vi "setCrosstalkThreshold.vi"(0 "connection ID":refnum<k5>, 1 "axis":i32, 2 "threshold":i32, 3 "slipphasetime":i32, 5 "error":errorcluster) -> (14 "connection ID out":refnum<k5>, 15 "axis_out":i32, 19 "error out":errorcluster)   [LabVIEW 2016, in "amc_api.lvlib"]
doc: "This function sets the threshold range to avoid axis-crosstalk and slip phase time which is used while moving another axis"
uses:
  amc_api.lvlib
panel:
  out "jsonRespIn":string
  out "JSON-response":string="{\"jsonrpc\":\"2.0\",\"method\":\"\",\"params\":[5,1.245,true,\"name\"],\"id\":\"1\"}"
  out "JSON request":string
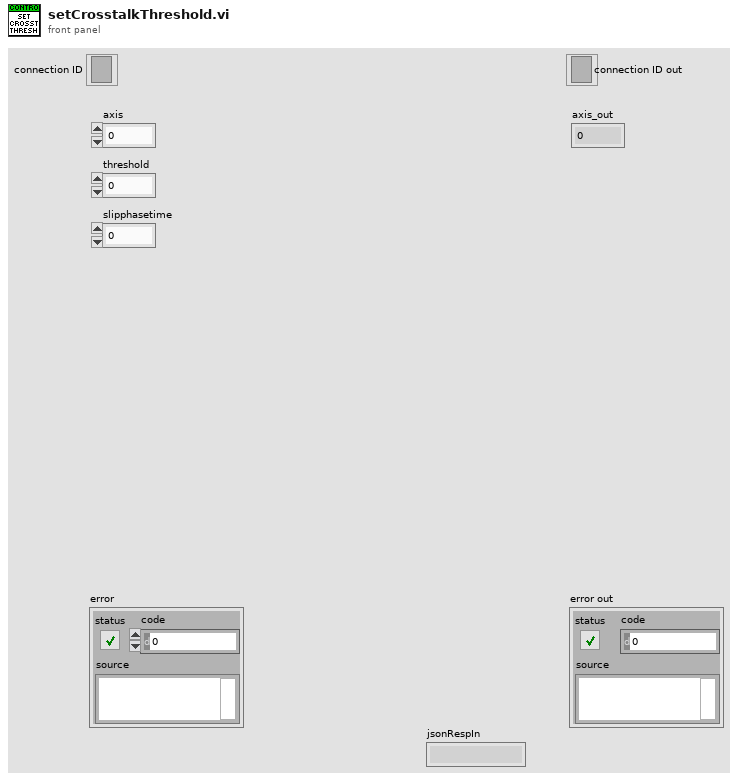
[diagram p1: front panel]
types:
  T1 = cluster{"jsonrpc":string, "method":string, "params":string[], "id":string, "api":i32, "pid":string}
  T2 = enum16{"Standard", "Buffered", "CRLF", "Immediate"}
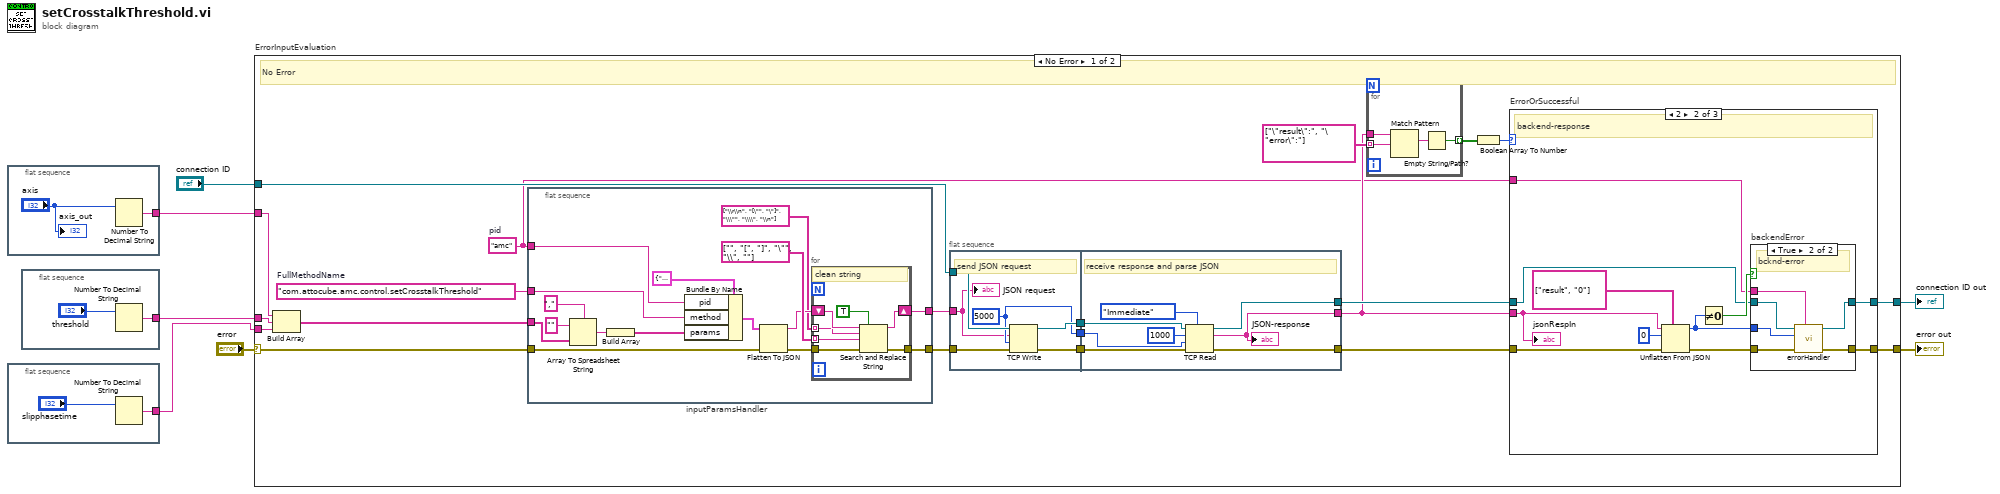
[diagram p0: block diagram]
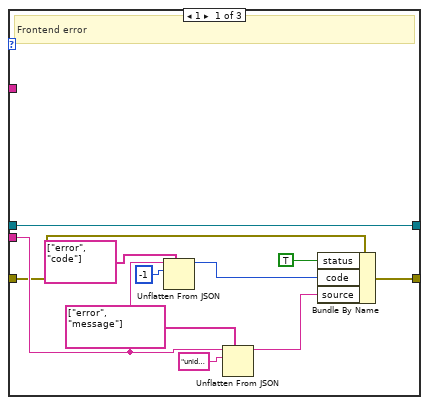
[diagram p2: hidden frame]
diagram:
  n1 = flat-sequence "in_axis" {
    tunnel: [w9] -> w3
    frame #0 {
      n2 = Number To Decimal String(number="axis") -> (decimal integer string=w9:string)  [unwired: 1 in]
      "axis_out" <- "axis"
    }
  }
  n3 = flat-sequence "in_integer" {
    tunnel: [w10] -> w1
    frame #0 {
      n4 = Number To Decimal String(number="slipphasetime") -> (decimal integer string=w10:string)  [unwired: 1 in]
    }
  }
  n5 = flat-sequence "in_integer" {
    tunnel: [w12] -> w2
    frame #0 {
      n6 = Number To Decimal String(number="threshold") -> (decimal integer string=w12:string)  [unwired: 1 in]
    }
  }
  n7 = case "ErrorInputEvaluation" shown="No Error" "error" {
    selector: "error" -> [w27 w108]
    tunnel: "connection ID" -> [w31 w109]
    tunnel: [w18 w108] -> w6
    tunnel: [w19 w109] -> w5
    tunnel: w3 -> [w16 _]
    tunnel: w2 -> [w15 _]
    tunnel: w1 -> [w14 _]
    frame No Error {
      w17 = "amc"  # pid
      w28 = "com.attocube.amc.control.setCrosstalkThreshold"  # FullMethodName
      # "No Error"
      n8 = Build Array ("ParametersArrayString")(w16, w15, w14) -> (w26:string[])
      n9 = flat-sequence "inputParamsHandler" {
        tunnel: [w72] -> w25
        tunnel: w26 -> [w78]
        tunnel: w27 -> [w77]
        tunnel: [w74] -> w24
        tunnel: w28 -> [w68]
        tunnel: w17 -> [w67]
        frame #0 {
          n10 = Array To Spreadsheet String(delimiter (Tab)=",", array=w78, 3:"" ("format string")) -> (spreadsheet string=w80:string)
          n11 = Build Array "Build Array"(w80) -> (w69:string[])
          n12 = Bundle By Name(cluster=T1 {"jsonrpc"="2.0", "method"="com.attocube.amc.res.setRESReadOutFreq", "params"=[], "id"="1", "api"=2, "pid"=""} ("Cluster"), "pid"=w67, "method"=w68, "params"=w69) -> (w79:T1)
          n13 = Flatten To JSON(anything=w79, error in (no error)=w77) -> (JSON string=w73:string, 11:w75:errorcluster)  [unwired: 1 in]
          n14 = for {
            tunnel: string[] ["\\r\\n", "[\"", "\"]", "\\\"", "\\\\", "\\n"] ("search string") -> [w86] mode=indexing
            tunnel: string[] ["", "[", "]", "\"", "\\", ""] ("replace string (\"\")") -> [w85] mode=indexing
            shift-right: [w88] -> w72
            shift-left: w73 -> [w87]
            tunnel: w75 -> [w84]
            tunnel: [w83] -> w74
            # "clean string"
            n15 = Search and Replace String(replace all?=TRUE ("replace all? (F)"), input string=w87, search string=w86, replace string=w85, error in=w84) -> (result string=w88:string, error out=w83:errorcluster)  [unwired: 3 in, 2 out]
          }
        }
      }
      n16 = flat-sequence {
        tunnel: w31 -> [w99]
        tunnel: [w97] -> w34
        tunnel: [w98] -> w33
        tunnel: w24 -> [w94]
        tunnel: [w96] -> w32
        tunnel: w25 -> [w95]
        tunnel: [w103] -> w23
        tunnel: w34 -> [w105]
        tunnel: w33 -> [w104]
        tunnel: [w101] -> w22
        tunnel: w32 -> [w102]
        tunnel: [w100] -> w21
        frame #0 {
          w96 = 5000 ("timeout ms (25000)")
          # "send JSON request"
          n17 = TCP Write(connection ID=w99, data in=w95, error in (no error)=w94, 9:w96) -> (connection ID out=w97:refnum<k5>, error out=w98:errorcluster)  [unwired: 1 out]
          "JSON request" <- w95
        }
        frame #1 {
          # "receive response and parse JSON"
          n18 = TCP Read(connection ID=w105, bytes to read=1000, error in (no error)=w104, 7:T2."Immediate" ("mode (standard)"), 9:w102) -> (connection ID out=w103:refnum<k5>, data out=w100:string, error out=w101:errorcluster)
          "JSON-response" <- w100
        }
      }
      n19 = for {
        tunnel: string[] ["\"result\":", "\"error\":"] ("path") -> [w92] mode=indexing
        tunnel: [w90] -> w29 mode=indexing
        tunnel: w21 -> [w93]
        n20 = Match Pattern(string=w93, regular expression=w92) -> (match substring=w91:string)  [unwired: 1 in, 3 out]
        n21 = Empty String/Path?(string/path=w91) -> (empty?=w90:bool)
      }
      n22 = Boolean Array To Number(Boolean array=w29) -> (number=w20:u32)
      n23 = case "ErrorOrSuccessful" shown="2" w20 {
        tunnel: w21 -> [w37 w48 _]
        tunnel: w23 -> [w35 w50 w66]
        tunnel: [w35 w49 w66] -> w19
        tunnel: [w38 w46 w65] -> w18
        tunnel: w22 -> [w36 w47 w65]
        tunnel: w17 -> [_ w51 _]
        frame 1 {
          # "Frontend error"
          n24 = Unflatten From JSON(path=string[] ["error", "code"], JSON string=w37, type and defaults=-1) -> (value=w44:i32)  [unwired: 4 in, 1 out]
          n25 = Unflatten From JSON(path=string[] ["error", "message"], JSON string=w37, type and defaults="unidentified error") -> (value=w45:string)  [unwired: 4 in, 1 out]
          n26 = Bundle By Name(cluster=w36, "status"=TRUE, "code"=w44, "source"=w45) -> (w38:errorcluster)
        }
        frame 2 {
          # "backend-response"
          n27 = Unflatten From JSON(path=string[] ["result", "0"], JSON string=w48, type and defaults=0, error in (no error)=w47) -> (value=w52:i32, error out=w54:errorcluster)  [unwired: 3 in]
          n28 = Not Equal To 0?(x=w52) -> (x != 0?=w53:bool)
          n29 = case "backendError" shown="True" w53 {
            tunnel: w52 -> [_ w64]
            tunnel: w54 -> [w58 w63]
            tunnel: [w57 w62] -> w49
            tunnel: [w58 w61] -> w46
            tunnel: w50 -> [w57 w60]
            tunnel: w51 -> [_ w59]
            frame False {
              # "successful"
            }
            frame True {
              # "bcknd-error"
              n30 = call "errorHandler.vi"("pid"=w59, "error in"=w63, "errNbr"=w64, "connection ID"=w60) -> ("error out 2"=w61:errorcluster, "connection ID out"=w62:refnum<k5>)  [unwired: 6 in]
            }
          }
          "jsonRespIn" <- w48
        }
        frame Default {
          # "NoResponse"
        }
      }
    }
    frame Error {
      # "Error"
    }
  }
  "error out" <- w6
  "connection ID out" <- w5
